vi "parser.vi"() -> ()   [LabVIEW 2009]
uses:
  <vilib>/Utility/file.llb/Read From Spreadsheet File (string).vi
  Global Test Variables DPT.vi
panel:
  out "Header":string[](array[string])
  out "all rows":string[][](array[string])
  out "File Data Out":string[][](array[string])
  in  "OK":bool
  out "array":string[][](array[string])
  out "search string":string
  out "Search for first column data":string
  in  "file path (dialog if empty)":path=path "c:/test1/test.csv"
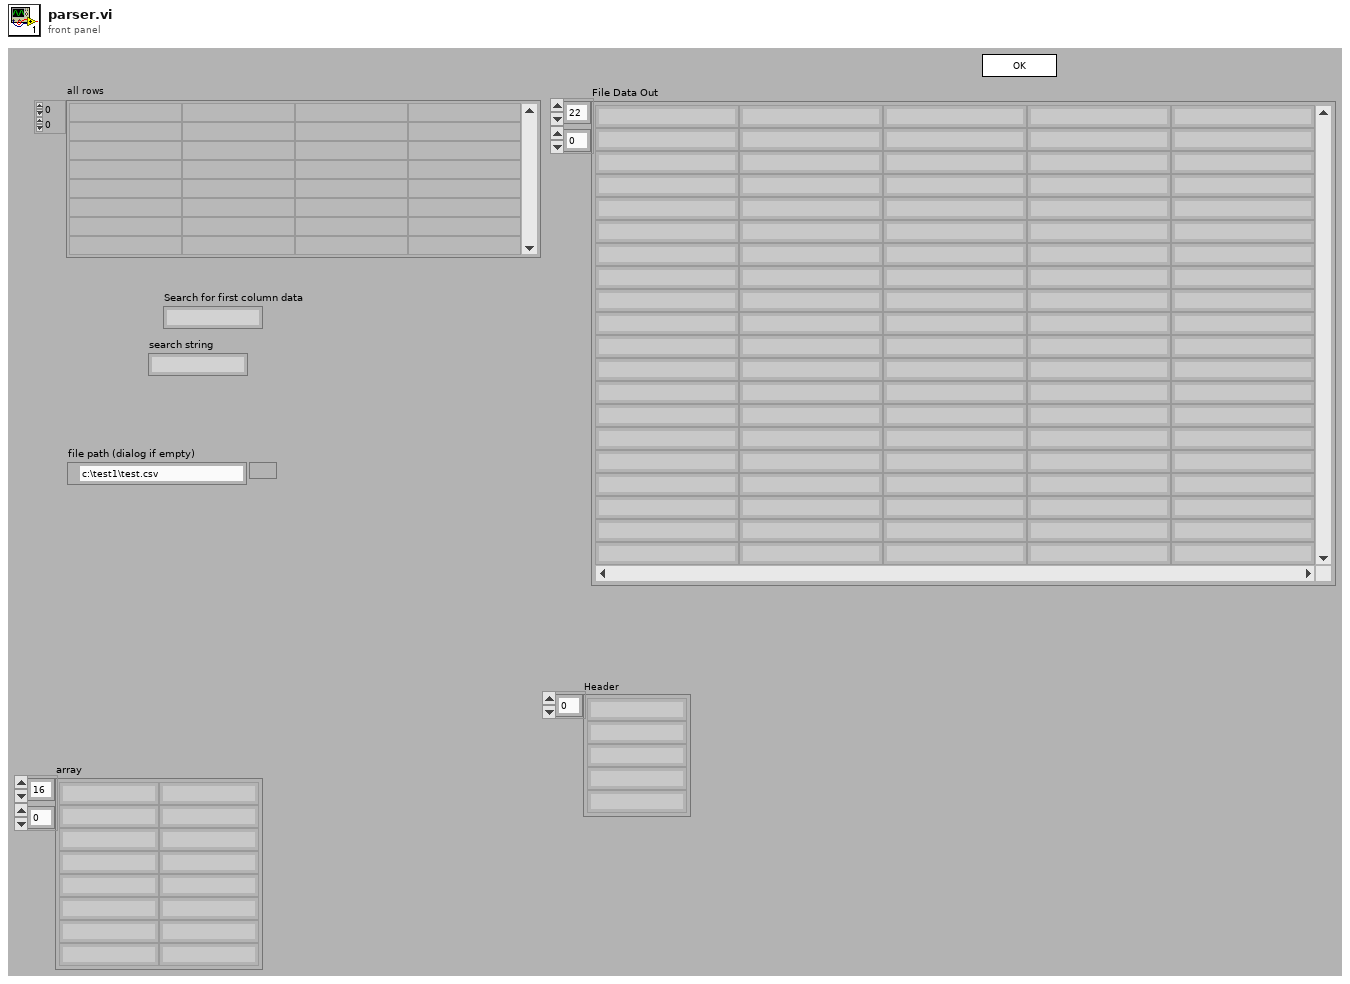
[diagram p1: front panel]
types:
  T1 = enum32{"invalid app kind", "Development System", "Run Time System", "Student Edition", "Embedded LabVIEW", "Evaluation", "Custom"}
  T2 = enum32{"Invalid", "Standard", "Closed", "Hidden", "Minimized", "Maximized"}
  T3 = cluster{"Core":cluster{"Current VI Reference":refnum<vi>, "Close Panel on Exit?":bool}, "File Data In":string[][], "file path (dialog if empty)":path, "File Data Out":string[][], "Header Labels":string[], "Data":dbl[][]}
  T4 = cluster{"Current VI Reference":refnum<vi>, "Close Panel on Exit?":bool}
  T5 = typedef "DOE Audit Data.ctl" = cluster{"Technician":string, "Date":string, "Model":string, "Serial":string, "Total Dry Time(m)":dbl, "Bone Dry Wt":dbl, "Initial Wt":dbl, "Final Wt":dbl, "Initial Ret":dbl, "Final Ret":dbl, "Elect Energy Used":dbl, "Gas Meter Temp":dbl, "Gas Meter Pres":dbl, "Gas Volume":dbl, "Barometer Temp":dbl, "Barometer Pres":dbl, "Gas Corr Fact":dbl, "Cor Gas Vol":dbl, "Gas Heat Val":dbl, "Gas Energy BTU":dbl, "Gas Energy kwh":dbl, "Total Energy":dbl, "4% adjust Energy":dbl, "Gas Vol Init":dbl, "Gas Vol Fin":dbl, "Start Time(s)":dbl, "End Time(s)":dbl, "Elect Energy Start":dbl, "Elect Energy End":dbl, "Per Cycle Efficency":dbl, "Annual Consumption":dbl, "Load Cycles":string, "Ambinet Temp":string, "Ambinet RH":string}
  T6 = cluster{"Initial Wt":dbl, "Final Wt":dbl, "Initial Ret":dbl, "Final Ret":dbl}
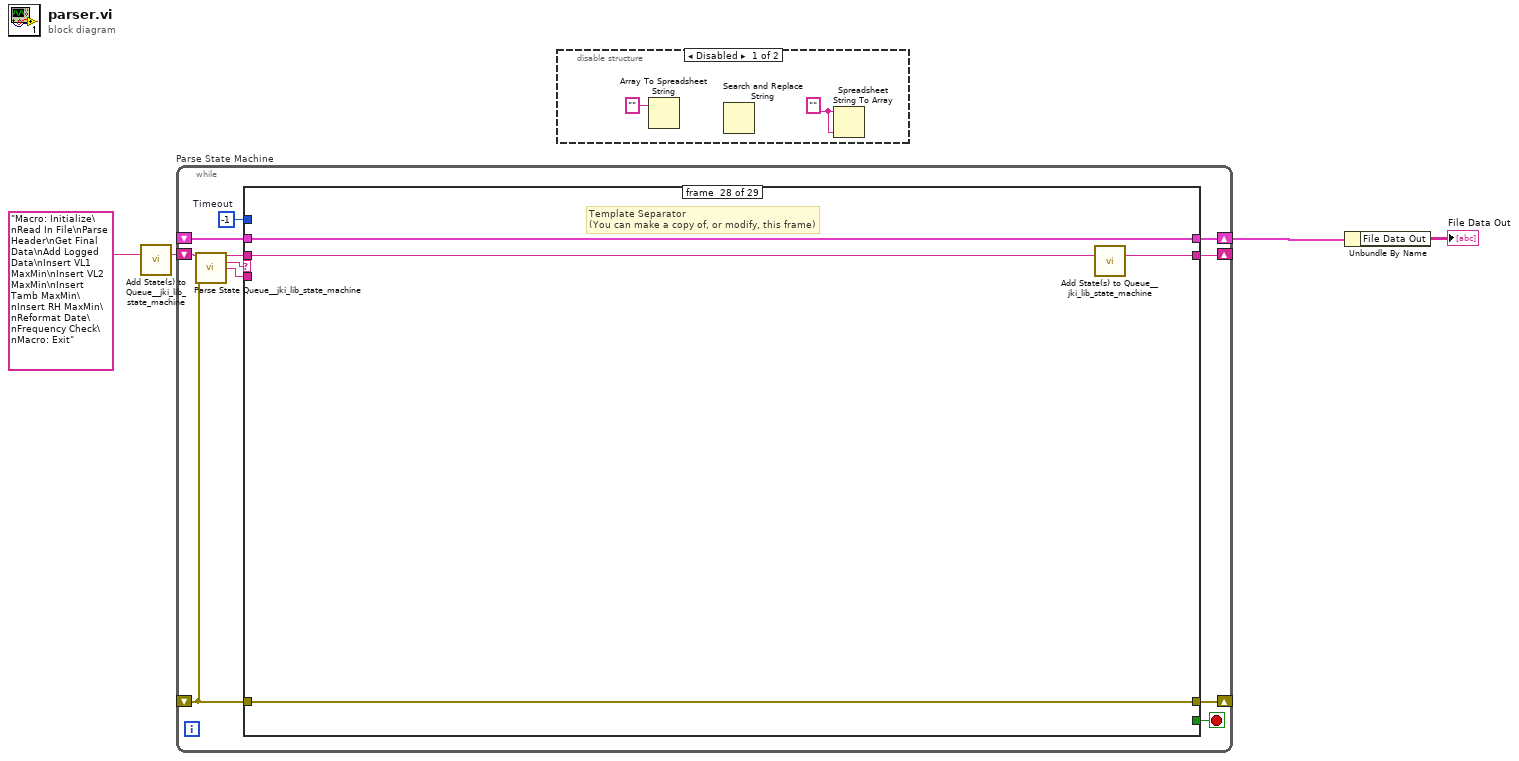
[diagram p0: block diagram]
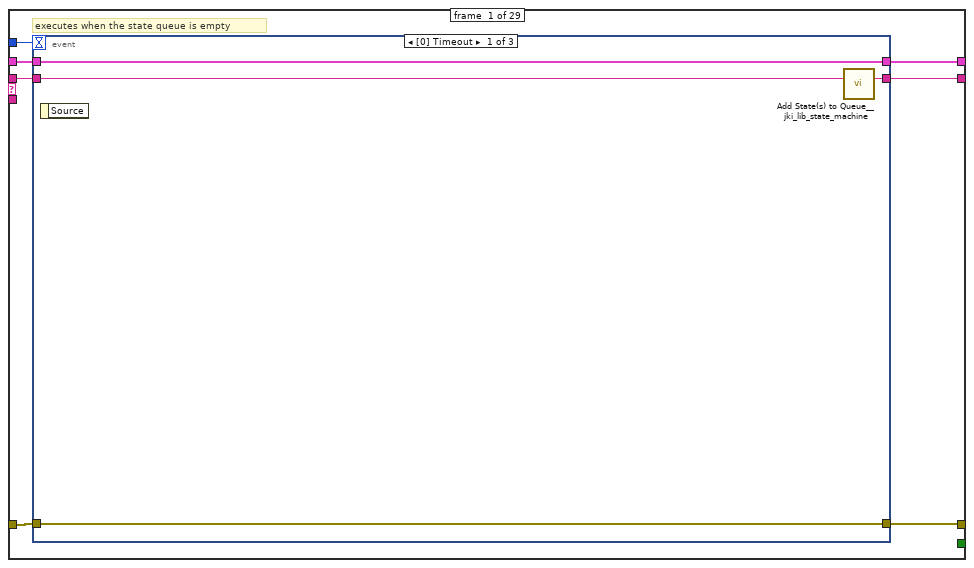
[diagram p3: hidden frame]
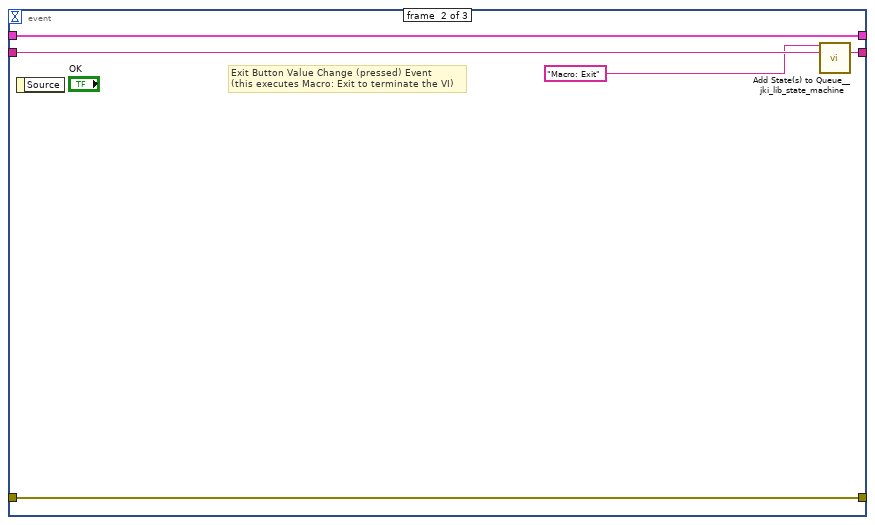
[diagram p4: hidden frame]
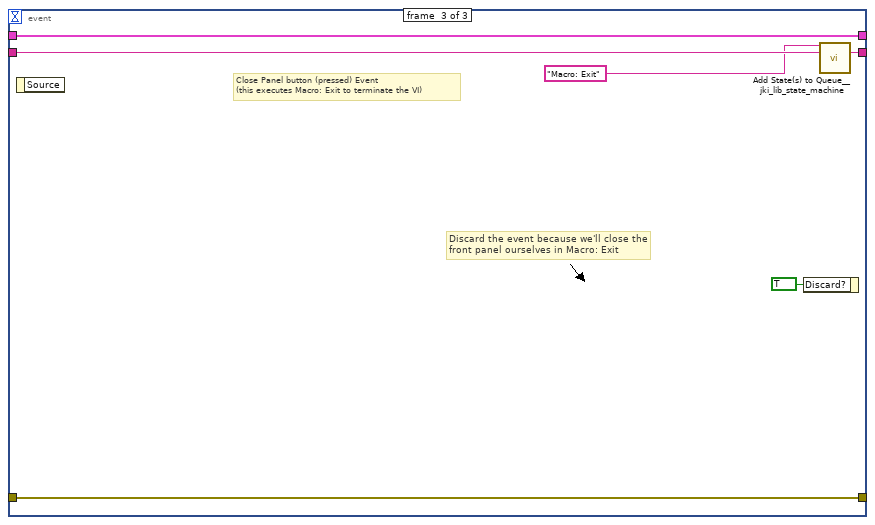
[diagram p5: hidden frame]
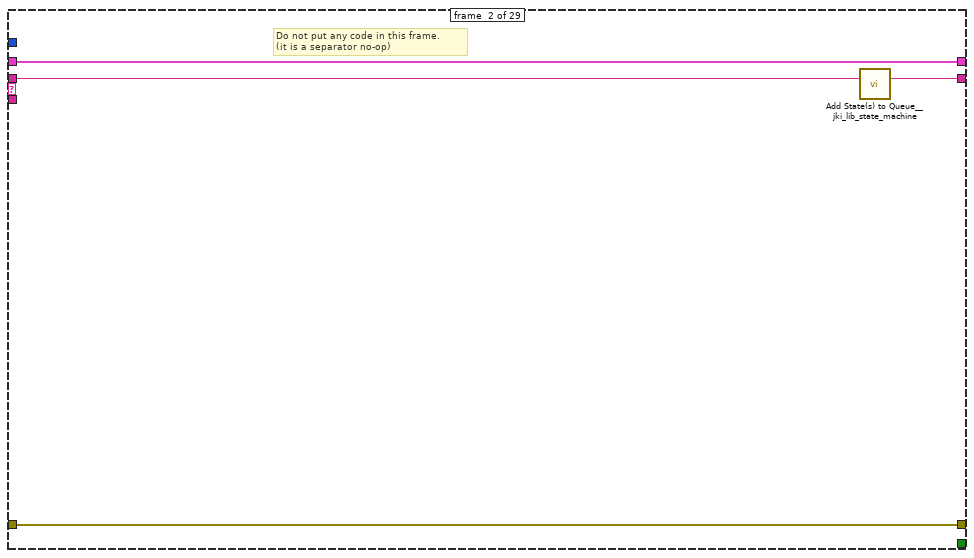
[diagram p6: hidden frame]
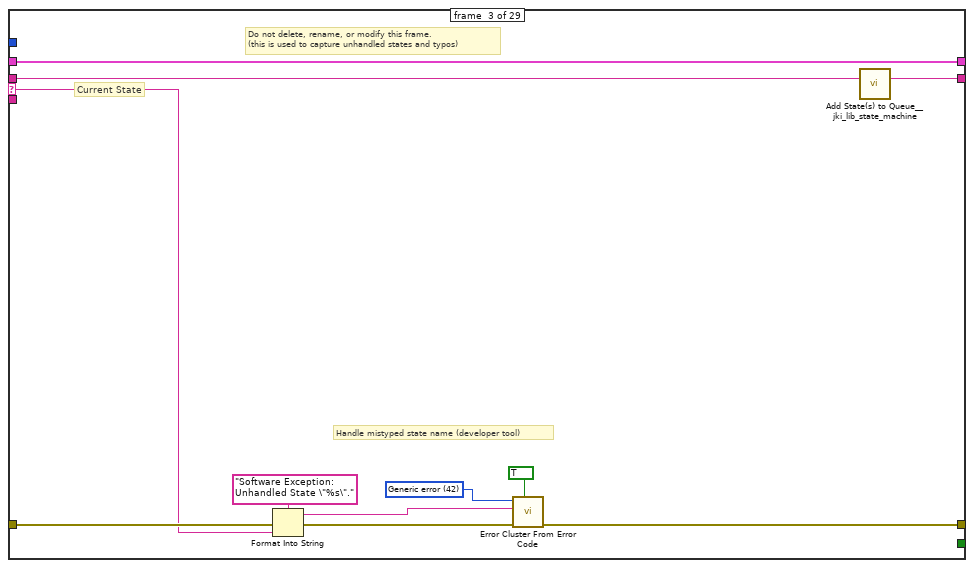
[diagram p7: hidden frame]
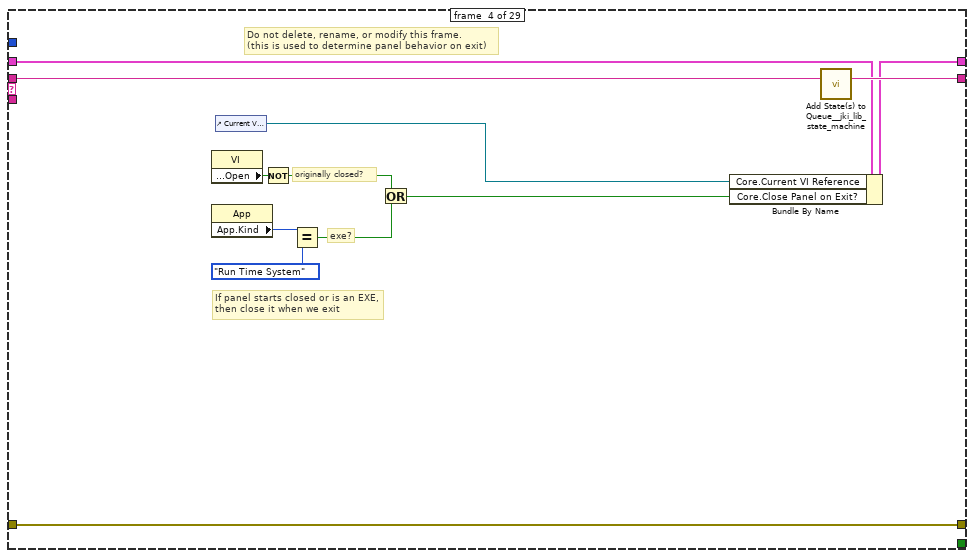
[diagram p8: hidden frame]
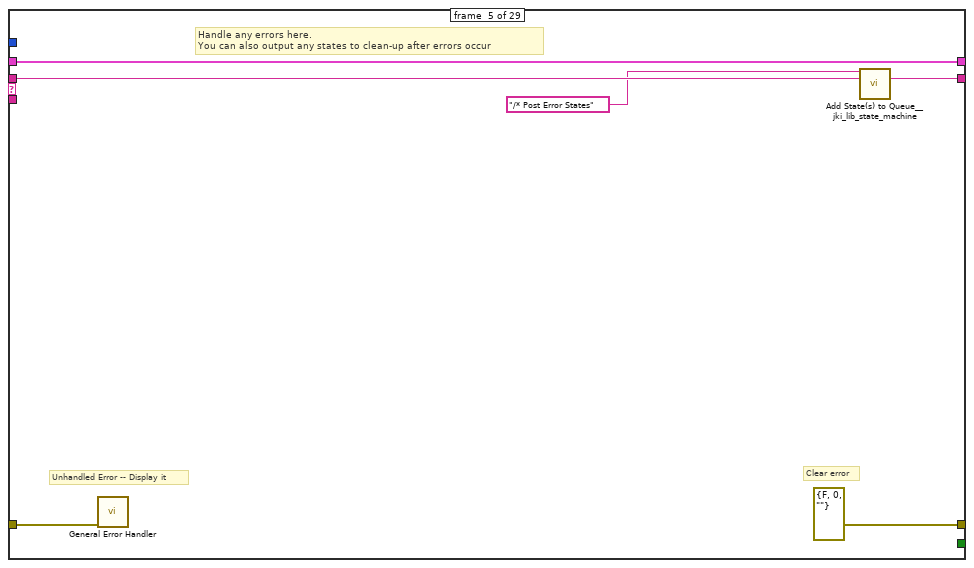
[diagram p9: hidden frame]
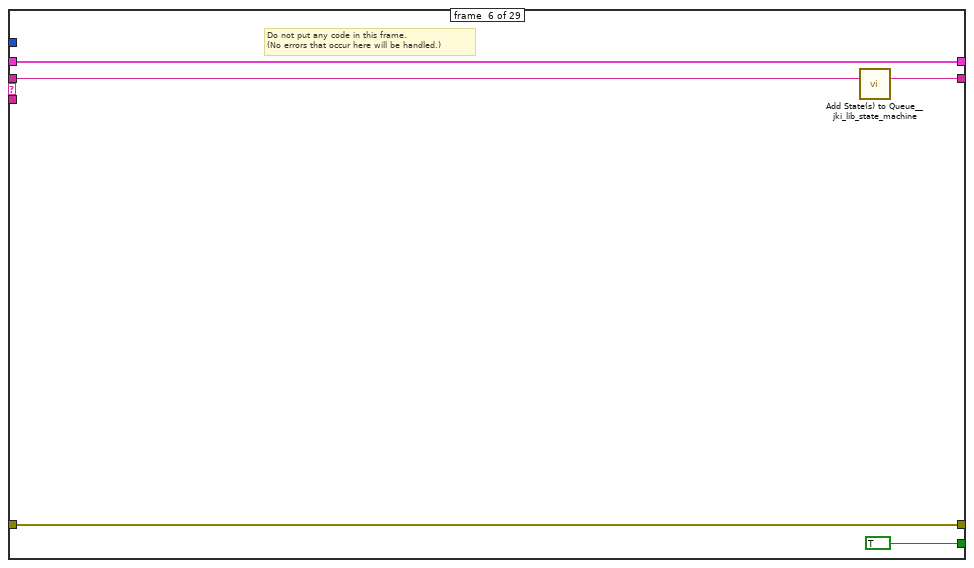
[diagram p10: hidden frame]
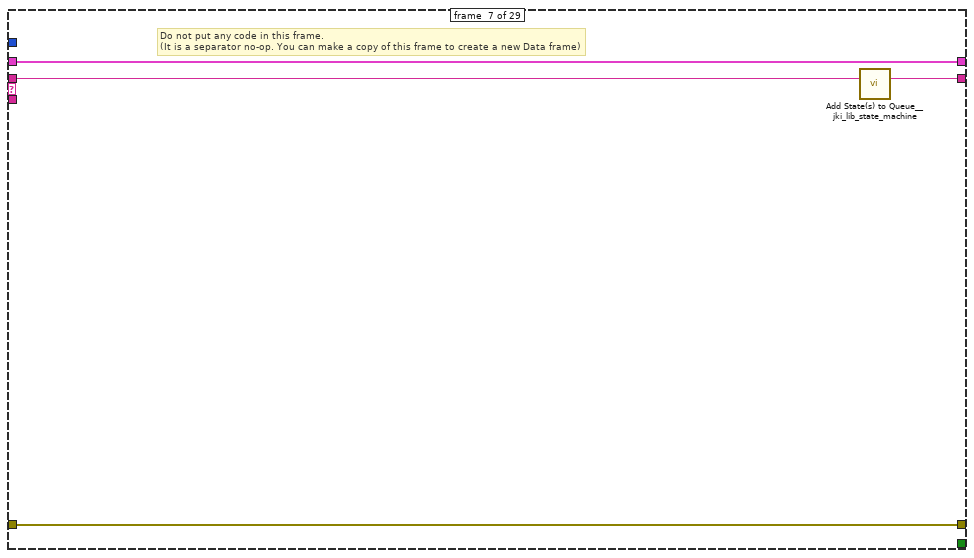
[diagram p11: hidden frame]
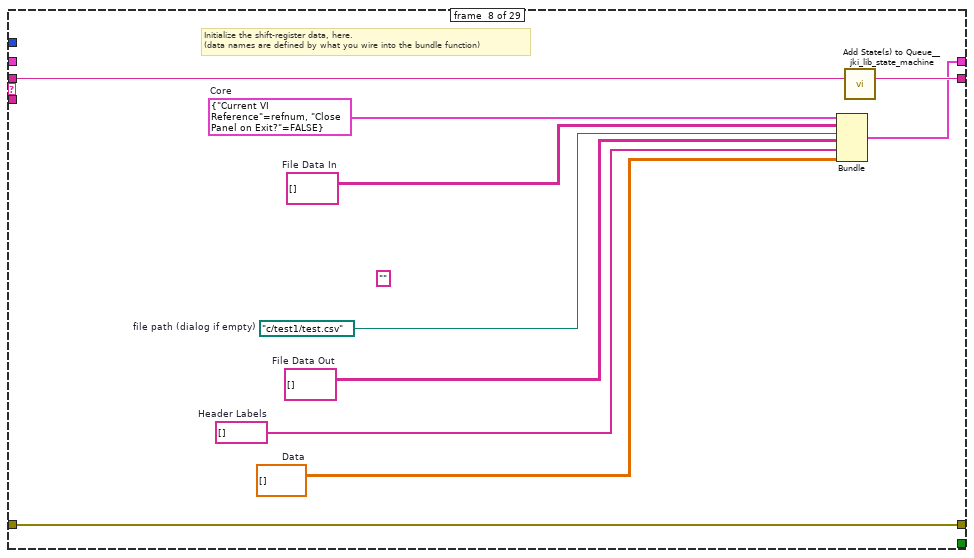
[diagram p12: hidden frame]
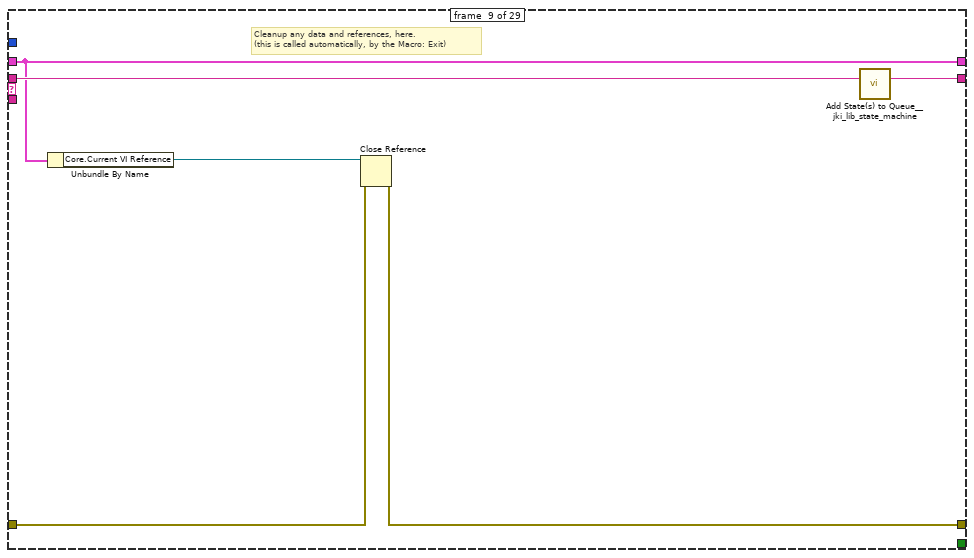
[diagram p13: hidden frame]
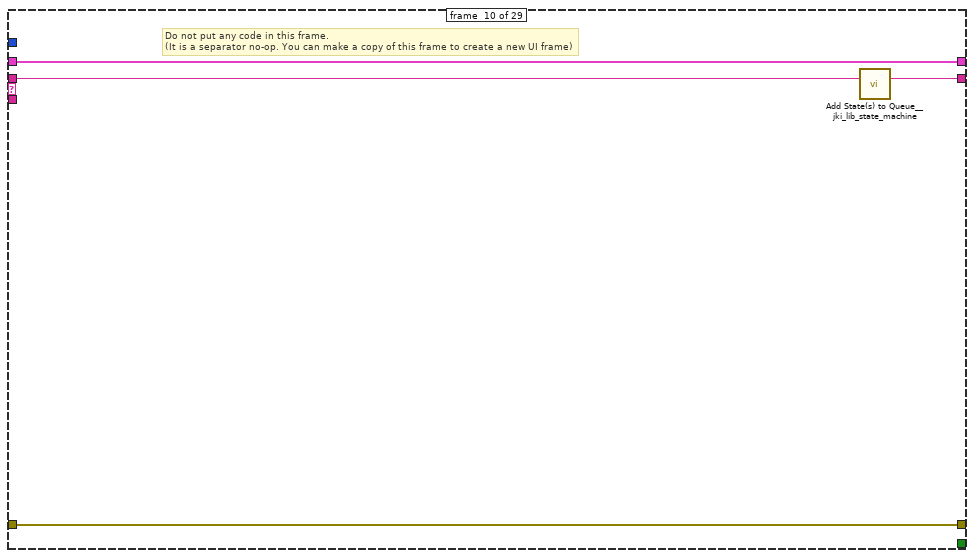
[diagram p14: hidden frame]
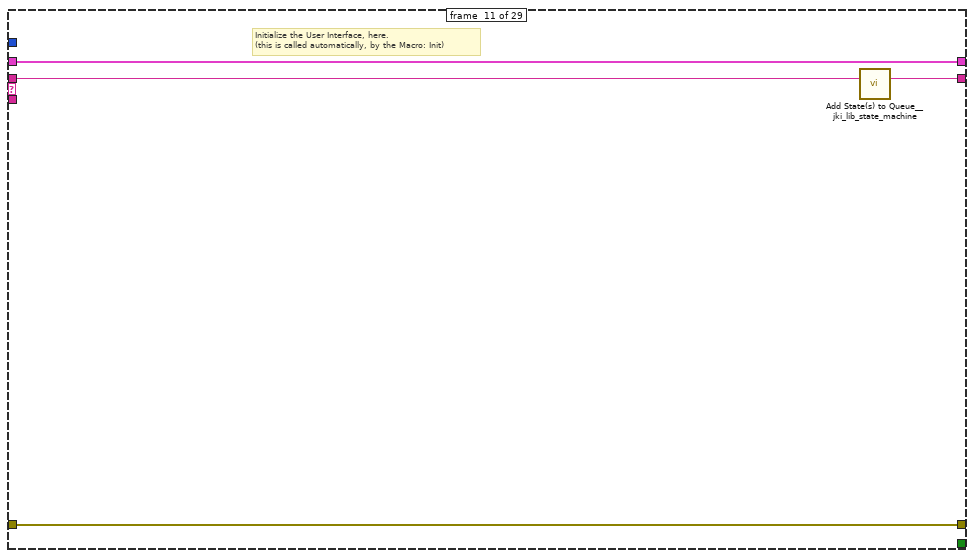
[diagram p15: hidden frame]
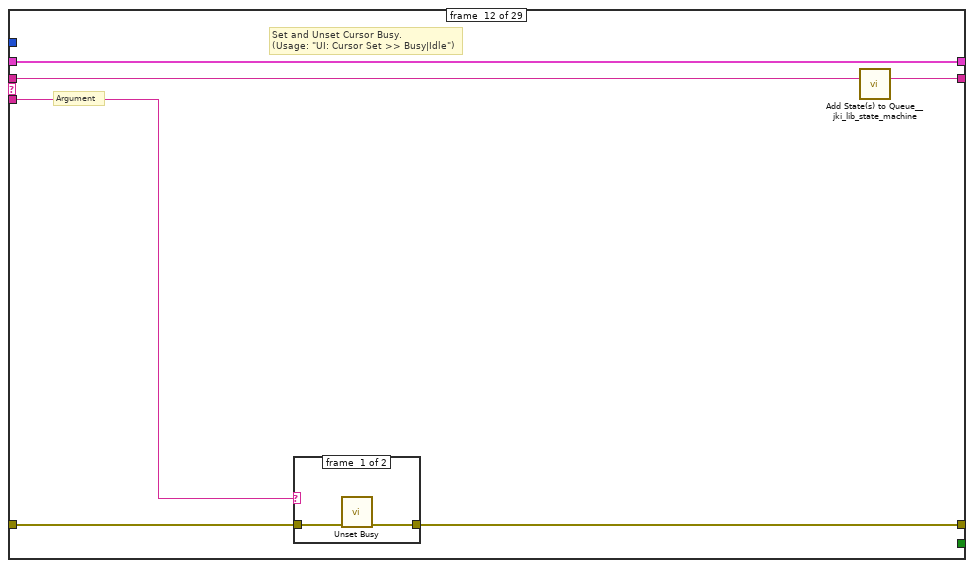
[diagram p16: hidden frame]
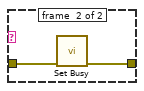
[diagram p17: hidden frame]
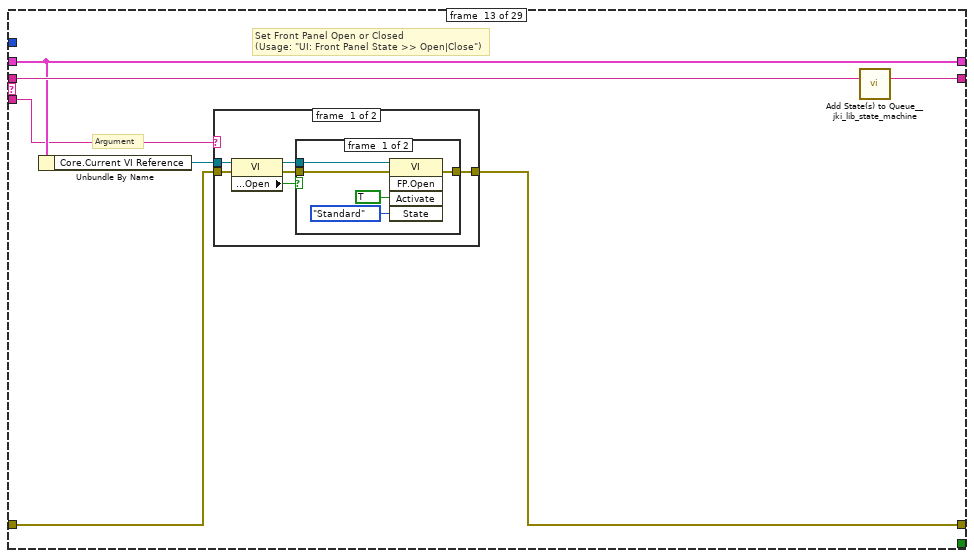
[diagram p18: hidden frame]
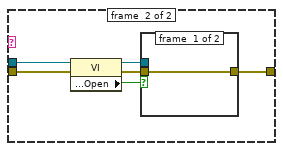
[diagram p20: hidden frame]
diagram:
  n1 = call <vilib>:"Add State(s) to Queue__jki_lib_state_machine.vi"("State(s) in (\"\")"="Macro: Initialize\nRead In File\nParse Header\nGet Final Data\nAdd Logged Data\nInsert VL1 MaxMin\nInsert VL2 MaxMin\nInsert Tamb MaxMin\nInsert RH MaxMin\nReformat Date\nFrequency Check\nMacro: Exit") -> ("States Out"=w4:string)  [unwired: 14 in]
  n2 = while "Parse State Machine" {
    shift-right: [w8] -> w2
    shift-left: _ -> [w7]
    shift-right: [w11] -> _
    shift-left: _ -> [w5]
    shift-right: [w10] -> _
    shift-left: w4 -> [w12]
    stop <- w9 stop-if-true
    w6 = -1  # Timeout
    n3 = call <vilib>:"Parse State Queue__jki_lib_state_machine.vi"("State Queue"=w12, "Error In (no error)"=w5) -> ("Remaining States"=w14:string, "Current State"=w15:string, "Arguments"=w13:string)  [unwired: 11 in]
    n4 = case shown="\"Get Final Data\"" w15 {
      selector: w15 -> [_ _ w42 _ _ _ _ _ _ _ _ _ _ _ _ _ _ _ _ _ _ _ _ _ _ _ _ _ _]
      tunnel: w14 -> [w22 w41 w46 w64 w70 w75 w79 w89 w95 w99 w103 w109 w120 w146 w151 w161 w165 w173 w190 w227 w249 w315 w341 w367 w393 w415 w430 w440 w454]
      tunnel: w13 -> [_ _ _ _ _ _ _ _ _ _ _ w104 w114 _ _ _ _ _ _ _ _ _ _ _ _ _ _ _ w444]
      tunnel: w7 -> [w20 w38 w44 w55 w67 w73 w76 _ w90 w96 w101 w107 w116 w143 w148 w158 w162 w168 w177 w212 w246 w297 w323 w349 w375 w395 w421 w437 w451]
      tunnel: [w19 w39 w48 w61 errorcluster {"status"=FALSE, "code"=0, "source"=""} ("error out") w72 w77 w86 w91 w97 w100 w105 w117 w144 w149 w159 w163 w171 w188 w225 w247 w313 w339 w365 w391 w413 w428 w438 w452] -> w11
      tunnel: w5 -> [w18 w39 w47 w61 w66 w72 w77 w86 w92 w97 w100 w106 w118 w144 w149 w159 w163 w171 w188 w225 w247 w313 w339 w365 w391 w413 w428 w438 w452]
      tunnel: [w21 w40 w45 w63 w69 w74 w78 w88 w94 w98 w102 w108 w119 w145 w150 w160 w164 w172 w189 w226 w248 w314 w340 w366 w392 w414 w429 w439 w453] -> w10
      tunnel: [_ _ _ _ _ TRUE _ _ _ _ _ _ _ _ _ _ _ _ _ _ _ _ _ _ _ _ _ _ _] -> w9
      tunnel: [w17 w38 w44 w62 w67 w73 w76 w87 w90 w96 w101 w107 w116 w143 w148 w158 w162 w167 w176 w211 w245 w297 w323 w349 w375 w396 w422 w437 w450] -> w8
      tunnel: w6 -> [w16 _ _ _ _ _ _ _ _ _ _ _ _ _ _ _ _ _ _ _ _ _ _ _ _ _ _ _ _]
      frame #0 {
        # "executes when the state queue is empty"
        n5 = event shown="[0] Timeout" {
          selector: _ -> [_ _ _]
          dyn-events: _ -> [_ _ _]
          timeout: w16 -> [_ _ _]
          tunnel: w22 -> [w26 w31 w37]
          tunnel: [w25 w30 w36] -> w21
          tunnel: w20 -> [w23 w28 w34]
          tunnel: [w24 w29 w35] -> w19
          tunnel: w18 -> [w24 w29 w35]
          tunnel: [w23 w28 w34] -> w17
          event #0 {
            n6 = event-data() -> ()  [unwired: 1 in, 1 out]
            n7 = call <vilib>:"Add State(s) to Queue__jki_lib_state_machine.vi"("State(s) in (\"\")"=w26) -> ("States Out"=w25:string)  [unwired: 14 in]
          }
          event #1 {
            # "Exit Button Value Change (pressed) Event\n(this executes Macro: Exit to terminate the VI)"
            n8 = event-data() -> ()  [unwired: 1 in, 1 out]
            n9 = call <vilib>:"Add State(s) to Queue__jki_lib_state_machine.vi"("State(s) in Front (\"\")"="Macro: Exit", "State(s) in (\"\")"=w31) -> ("States Out"=w30:string)  [unwired: 13 in]
          }
          event #2 {
            # "Discard the event because we'll close the front panel ourselves in Macro: Exit"
            # "Close Panel button (pressed) Event\n(this executes Macro: Exit to terminate the VI)"
            n10 = event-data() -> ()  [unwired: 1 in, 1 out]
            n11 = event-data("Discard?"=TRUE) -> ()  [unwired: 1 in, 1 out]
            n12 = call <vilib>:"Add State(s) to Queue__jki_lib_state_machine.vi"("State(s) in Front (\"\")"="Macro: Exit", "State(s) in (\"\")"=w37) -> ("States Out"=w36:string)  [unwired: 13 in]
          }
        }
      }
      frame #1 {
        # "Do not put any code in this frame.\n(it is a separator no-op)"
        n13 = call <vilib>:"Add State(s) to Queue__jki_lib_state_machine.vi"("State(s) in (\"\")"=w41) -> ("States Out"=w40:string)  [unwired: 14 in]
      }
      frame #2 {
        w51 = 42 items=["No error", "Argument error", "Memory is full", "Out of zone", "End of file", "File already open", "Generic file I/O error", "File not found", "File permission error", "Disk is full", "Duplicate path", "Too many files open", "System feature not enabled", "Resource file not found", "Cannot add resource", "Resource not found", "Image not found", "Image memory error", "Pen does not exist", "Config type invalid", "Config token not found", "Config parse error", "Config memory error", "Bad external code format", "Bad external code offset", "External code not present", "Null window", "Destroy window error", "Null menu", "Print aborted", "Bad print record", "Print driver error", "Windows error during printing", "Memory error during printing", "Print dialog error", "Generic print error", "Invalid device refnum", "Device not found", "Device parameter error", "Device unit error", "Cannot open device", "Device call aborted", "Generic error", "Cancelled by user", "Object ID too low", "Object ID too high", "Object not in heap", "Unknown heap", "Unknown object (invalid DefProc)", "Unknown object (DefProc not in table)", "Message out of range", "Invalid (null) method", "Unknown message", "Manager call not supported", "Bad address", "Network operation in progress", "Network operation timed out", "Connection is busy", "Network attribute not supported", "Network error", "Address in use", "System out of memory", "Connection aborted", "Connection refused", "Not connected", "Already connected", "Connection closed", "Initialization error (interapplication manager)", "Bad occurrence", "Wait on unbound occurrence handler", "Occurrence queue overflow", "Datalog type conflict", "Unused", "Unrecognized type (interapplication manager)", "Memory corrupt", "Failed to make temporary DLL", "Old CIN version", "Drag socket not found", "Failed to load drop-object", "Failed to register OLE object", "Failed to release OLE object", "Format specifier type mismatch", "Unknown format specifier", "Too few format specifiers", "Too many format specifiers", "Scan failed", "Newer CIN version", "Error converting to variant", "Runtime menu error", "Password tampered", "Variant attribute not found", "Incompatible variant data type", "Event data is not available", "Event Store is not present", "Occurrence is not found", "Event Queue is not created", "Event info is not available", "Refnum passed is NULL", "Error retrieving Class GUID", "Error retrieving CoClass GUID", "Error retrieving TypeLib GUID.", "Bad built application magic bytes.", "Specific driver is different from the specific driver associated with the Logical Name.", "There is no session opened to the class driver.", "Max Error", "MAX - Error with config objects", "MAX - Error loading configuration", "MAX - Group not supported"]
        # "Current State"
        # "Do not delete, rename, or modify this frame.\n(this is used to capture unhandled states and typos)"
        # "Handle mistyped state name (developer tool)"
        n14 = Format Into String(format string="Software Exception: Unhandled State \"%s\"." ("message"), error in=w47, w42) -> (resulting string=w50:string, error out=w49:errorcluster)  [unwired: 1 in]
        n15 = call <vilib>:"Error Cluster From Error Code.vi"("show call chain? (False)"=TRUE, "error in (no error)"=w49, "error message (\"\")"=w50, "error code (0)"=w51) -> ("error out"=w48:errorcluster)  [unwired: 5 in]
        n16 = call <vilib>:"Add State(s) to Queue__jki_lib_state_machine.vi"("State(s) in (\"\")"=w46) -> ("States Out"=w45:string)  [unwired: 14 in]
      }
      frame #3 {
        # "Do not delete, rename, or modify this frame.\n(this is used to determine panel behavior on exit)"
        # "originally closed?"
        # "exe?"
        # "If panel starts closed or is an EXE, then close it when we exit"
        n17 = property class="VI"() -> ("Front Panel.Open"=w60:bool)  [unwired: 2 in, 2 out]
        n18 = property class="App"() -> ("App.Kind"=w59:T1)  [unwired: 2 in, 2 out]
        n19 = control-ref of="Current VI Reference"() -> (w53:refnum<vi>)
        n20 = Not(x=w60) -> (.not. x?=w57:bool)
        n21 = Equal?(x=w59, y=T1."Run Time System" ("Application:Kind")) -> (x = y?=w56:bool)
        n22 = Or(x=w57, y=w56) -> (x .or. y?=w54:bool)
        n23 = Bundle By Name(cluster=w55, "Core.Current VI Reference"=w53, "Core.Close Panel on Exit?"=w54) -> (w62:T3)
        n24 = call <vilib>:"Add State(s) to Queue__jki_lib_state_machine.vi"("State(s) in (\"\")"=w64) -> ("States Out"=w63:string)  [unwired: 14 in]
      }
      frame #4 {
        # "Unhandled Error -- Display it"
        # "Handle any errors here.\nYou can also output any states to clean-up after errors occur"
        # "Clear error"
        n25 = call <vilib>:"General Error Handler.vi"("error in (no error)"=w66) -> ()  [unwired: 10 in, 5 out]
        n26 = call <vilib>:"Add State(s) to Queue__jki_lib_state_machine.vi"("State(s) in Front (\"\")"="/* Post Error States", "State(s) in (\"\")"=w70) -> ("States Out"=w69:string)  [unwired: 13 in]
      }
      frame #5 {
        # "Do not put any code in this frame.\n(No errors that occur here will be handled.)"
        n27 = call <vilib>:"Add State(s) to Queue__jki_lib_state_machine.vi"("State(s) in (\"\")"=w75) -> ("States Out"=w74:string)  [unwired: 14 in]
      }
      frame #6 {
        # "Do not put any code in this frame.\n(It is a separator no-op. You can make a copy of this frame to create a new Data frame)"
        n28 = call <vilib>:"Add State(s) to Queue__jki_lib_state_machine.vi"("State(s) in (\"\")"=w79) -> ("States Out"=w78:string)  [unwired: 14 in]
      }
      frame #7 {
        (unwired) "" ("String")
        w80 = dbl[][] []  # Data
        w81 = string[] []  # Header Labels
        w82 = string[][] []  # File Data Out
        w83 = path "c:/test1/test.csv"  # file path (dialog if empty)
        w84 = string[][] []  # File Data In
        w85 = T4 {"Current VI Reference"=refnum, "Close Panel on Exit?"=FALSE}  # Core
        # "Initialize the shift-register data, here.\n(data names are defined by what you wire into the bundle function)"
        n29 = Bundle("Core"=w85, "File Data In"=w84, "file path (dialog if empty)"=w83, "File Data Out"=w82, "Header Labels"=w81, "Data"=w80) -> (w87:T3)  [unwired: 1 in]
        n30 = call <vilib>:"Add State(s) to Queue__jki_lib_state_machine.vi"("State(s) in (\"\")"=w89) -> ("States Out"=w88:string)  [unwired: 14 in]
      }
      frame #8 {
        # "Cleanup any data and references, here.\n(this is called automatically, by the Macro: Exit)"
        n31 = Unbundle By Name(w90) -> ("Core.Current VI Reference"=w93:refnum<vi>)
        n32 = Close Reference(reference=w93, error in (no error)=w92) -> (error out=w91:errorcluster)
        n33 = call <vilib>:"Add State(s) to Queue__jki_lib_state_machine.vi"("State(s) in (\"\")"=w95) -> ("States Out"=w94:string)  [unwired: 14 in]
      }
      frame #9 {
        # "Do not put any code in this frame.\n(It is a separator no-op. You can make a copy of this frame to create a new UI frame)"
        n34 = call <vilib>:"Add State(s) to Queue__jki_lib_state_machine.vi"("State(s) in (\"\")"=w99) -> ("States Out"=w98:string)  [unwired: 14 in]
      }
      frame #10 {
        # "Initialize the User Interface, here.\n(this is called automatically, by the Macro: Init)"
        n35 = call <vilib>:"Add State(s) to Queue__jki_lib_state_machine.vi"("State(s) in (\"\")"=w103) -> ("States Out"=w102:string)  [unwired: 14 in]
      }
      frame #11 {
        # "Argument"
        # "Set and Unset Cursor Busy.\n(Usage: \"UI: Cursor Set >> Busy|Idle\")"
        n36 = case shown="\"Idle\", Default" w104 {
          tunnel: w106 -> [w111 w113]
          tunnel: [w110 w112] -> w105
          frame #0 {
            n37 = call <vilib>:"Unset Busy.vi"("error in (no error)"=w111) -> ("error out"=w110:errorcluster)  [unwired: 10 in]
          }
          frame #1 {
            n38 = call <vilib>:"Set Busy.vi"("error in (no error)"=w113) -> ("error out"=w112:errorcluster)  [unwired: 9 in, 1 out]
          }
        }
        n39 = call <vilib>:"Add State(s) to Queue__jki_lib_state_machine.vi"("State(s) in (\"\")"=w109) -> ("States Out"=w108:string)  [unwired: 14 in]
      }
      frame #12 {
        # "Argument"
        # "Set Front Panel Open or Closed\n(Usage: \"UI: Front Panel State >> Open|Close\")"
        n40 = Unbundle By Name(w116) -> ("Core.Current VI Reference"=w115:refnum<vi>)
        n41 = case shown="\"Open\", Default" w114 {
          tunnel: w118 -> [w124 w137]
          tunnel: [w126 w138] -> w117
          tunnel: w115 -> [w125 w135]
          frame #0 {
            n42 = property class="VI"(reference=w125, error in=w124) -> (reference out=w122:refnum<vi>, error out=w123:errorcluster, "Front Panel.Open"=w121:bool)
            n43 = case shown="False" w121 {
              tunnel: [w129 w132] -> w126
              tunnel: w123 -> [w128 w132]
              tunnel: w122 -> [w127 _]
              frame #0 {
                n44 = invoke class="VI" method="FP.Open"(reference=w127, error in=w128, "Activate"=TRUE, "State"=T2."Standard") -> (error out=w129:errorcluster)  [unwired: 1 in, 4 out]
              }
              frame #1 {
              }
            }
          }
          frame #1 {
            n45 = property class="VI"(reference=w135, error in=w137) -> (reference out=w134:refnum<vi>, error out=w136:errorcluster, "Front Panel.Open"=w133:bool)
            n46 = case shown="True" w133 {
              tunnel: [w139 w142] -> w138
              tunnel: w136 -> [w139 w141]
              tunnel: w134 -> [_ w140]
              frame #0 {
              }
              frame #1 {
                n47 = invoke class="VI" method="FP.Close"(reference=w140, error in=w141) -> (error out=w142:errorcluster)  [unwired: 1 in, 2 out]
              }
            }
          }
        }
        n48 = call <vilib>:"Add State(s) to Queue__jki_lib_state_machine.vi"("State(s) in (\"\")"=w120) -> ("States Out"=w119:string)  [unwired: 14 in]
      }
      frame #13 {
        # "Do not put any code in this frame.\n(It is a separator no-op. You can make a copy of this frame to create a new Macro frame)"
        n49 = call <vilib>:"Add State(s) to Queue__jki_lib_state_machine.vi"("State(s) in (\"\")"=w146) -> ("States Out"=w145:string)  [unwired: 14 in]
      }
      frame #14 {
        w147 = "Data: Initialize\nInitialize Core Data\nUI: Initialize\nUI: Front Panel State >> Open"  # Data: Initialize Initialize Core Data UI: Initialize UI: Front Panel State >> Open
        # "Initialization Macro\n(This is called once, when the VI starts)"
        n50 = call <vilib>:"Add State(s) to Queue__jki_lib_state_machine.vi"("State(s) in Front (\"\")"=w147, "State(s) in (\"\")"=w151) -> ("States Out"=w150:string)  [unwired: 13 in]
      }
      frame #15 {
        # "Exit Macro\n(This is called once, when the VI exits)"
        n51 = Unbundle By Name(w158) -> ("Core.Close Panel on Exit?"=w157:bool)
        n52 = Select(t="UI: Front Panel State >> Close", s=w157, f="") -> (s? t:f=w154:string)
        n53 = call <vilib>:"Add State(s) to Queue__jki_lib_state_machine.vi"("State(s) in (\"\")"=w154, "State(s) at Back (\"\")"="Data: Cleanup\nExit") -> ("States Out"=w152:string)  [unwired: 13 in]
        n54 = call <vilib>:"Add State(s) to Queue__jki_lib_state_machine.vi"("State(s) in Front (\"\")"=w152, "State(s) in (\"\")"=w161) -> ("States Out"=w160:string)  [unwired: 13 in]
      }
      frame #16 {
        # "Template Separator\n(You can make a copy of, or modify, this frame)"
        n55 = call <vilib>:"Add State(s) to Queue__jki_lib_state_machine.vi"("State(s) in (\"\")"=w165) -> ("States Out"=w164:string)  [unwired: 14 in]
      }
      frame #17 {
        n56 = call-poly <vilib>:"Read From Spreadsheet File.vi"("delimiter (\\t)"="," ("delimiter (\\t)"), "file path (dialog if empty)"="file path (dialog if empty)") -> ("all rows"=w166:string[][])  [unwired: 5 in, 4 out]
        "all rows" <- w166
        n57 = Bundle By Name(cluster=w168, "File Data In"=w166) -> (w167:T3)
        n58 = call <vilib>:"Add State(s) to Queue__jki_lib_state_machine.vi"("State(s) in (\"\")"=w173) -> ("States Out"=w172:string)  [unwired: 14 in]
      }
      frame #18 {
        w178 = "TEST STATION:\t&Station \nCOMPUTER_NAME:\t&Computername\nVERSION:\t&Version\nTR_NUMBER:\t&TR#\nENGINEER:\t&Engineer\nTECHNICIAN:\t&Tech\nFILENAME:\t&Filename\nCOMMENTS:\t&Comments\nDATE:\t&Date\nBuild\t&Build\nLAB ID:\t&Unit\nMODEL:\t&Model\nSerial Number\t&Serial\nSerial Number\t&Dryer Type\nSUPPLY VOLTAGE:\t&Voltage\nFrequency:\t&Freq\nDrum Volume\t&Volume\nTEST_TYPE:\t&Test Type\nTEST_TITLE:\t&Title\nTEST NUM:\t&Test Number\nNom Load Type\t&Load Type\nNom Load Weight\t&Load Size\nLOAD RUN NUM:\t&Run\nDRYING CYCLE:\t&Drying Cycle\nHeat Setting\t&Heat Setting\nDryness Setting\t&Dryness setting\nEXHAUST:\t&Restriction\nBone Dry Wt\t&BDW\n"  # Label, replace string
        w187 = "" ("format string")
        w179 = "" ("format string")
        w184 = "STATION / NAME:\t&Station / &Computername\nVERSION:\t&Version\n--------------------------\t--------------------------\nTR #:\t&TR#\nENGINEER:\t&Engineer\nTECHNICIAN:\t&Tech\n--------------------------\t--------------------------\nFILENAME:\t&Filename\nCOMMENTS:\t&Comments\nDATE:\t&Date\n--------------------------\t--------------------------\nBUILD:\t&Build\nUNIT:\t&Unit\nMODEL #:\t&Model\nSERIAL #:\t&Serial\nDRYER TYPE:\t&Dryer Type\nSUPPLY VOLTAGE:\t&Voltage\nFREQUENCY (Hz):\t&Freq\nDRUM VOL (cuft):\t&Volume\n--------------------------\t--------------------------\nTEST TYPE:\t&Test Type\nTEST TITLE:\t&Title\nTEST #:\t&Test Numver\nLOAD TYPE:\t&Load Type\nLOAD SIZE (lbs):\t&Load Size\nLOAD RUN #:\t&Run\n--------------------------\t--------------------------\nDRYING CYCLE:\t&Drying Cycle\nHEAT SETTING:\t&Heat Setting\nDRYNESS SETTING:\t&Dryness setting\nRESTRICTION:\t&Restriction\nBONE DRY WT (lbs):\t&BDW\nINITIAL WT (lbs):\t&InitWeight\nFINAL WT (lbs):\t&FinalWeight\nIMC:\t&IMC\nFMC:\t&FMC\nFMC DELAY (min):\t&FMCDelay\n--------------------------\t--------------------------\nAMB TEMP (F):\t&AmbTemp\nAMB RH (%):\t&RH\nAMB TEMP (Max / Min):\t&TempMaxMin\nAMB RH (Max / Min):\t&RHMaxMin\nVOLTAGE L1 (Max / Min):\t&VL1MaxMin\nVOLTAGE L2 (Max / Min):\t&VL2MaxMin\n--------------------------\t--------------------------\n"  # ProtoData
        # "Your code here.\n(You can make a copy of, or modify, this frame)"
        n59 = Unbundle By Name(w177) -> ("File Data In"=w175:string[][])
        n60 = local write "File Data Out"(w175) -> ()
        n61 = Delete From Array(array=w175, index (col)=0 ("disabled index (col)")) -> (deleted portion=w181:string[])  [unwired: 2 in, 1 out]
        n62 = Delete From Array(array=w175, index (col)=1 ("disabled index (col)")) -> (deleted portion=w183:string[])  [unwired: 2 in, 1 out]
        n63 = Spreadsheet String To Array(format string=w179, spreadsheet string=w178, array type (2D Dbl)=w179) -> (array=w185:string[][])  [unwired: 1 in]
        "array" <- w185
        n64 = for {
          tunnel: w181 -> [w201]
          tunnel: w183 -> [w199]
          tunnel: w185 -> [w196] mode=indexing
          shift-right: [w191] -> w186
          shift-left: w184 -> [w198]
          n65 = Index Array(array=w196, index #1=0 ("index"), index #2=1 ("index")) -> (element #1=w193:string, element #2=w192:string)
          "Search for first column data" <- w193
          "search string" <- w192
          n66 = Search 1D Array(1D array=w201, element=w193) -> (index of element=w200:i32)  [unwired: 1 in]
          n67 = Index Array(array=w199, index=w200) -> (element=w197:string)
          n68 = Search and Replace String(input string=w198, search string=w192, replace string=w197) -> (result string=w191:string)  [unwired: 5 in, 3 out]
        }
        n69 = Spreadsheet String To Array(format string=w187, spreadsheet string=w186, array type (2D Dbl)=w187) -> (array=w174:string[][])  [unwired: 1 in]
        n70 = Bundle By Name(cluster=w177, "File Data Out"=w174) -> (w176:T3)
        n71 = local write "File Data Out"(w174) -> ()
        n72 = call <vilib>:"Add State(s) to Queue__jki_lib_state_machine.vi"("State(s) in (\"\")"=w190) -> ("States Out"=w189:string)  [unwired: 14 in]
      }
      frame #19 {
        w206 = "" ("format string")
        # "Your code here.\n(You can make a copy of, or modify, this frame)"
        n73 = call "Worksheet DOE Audit.vi"() -> ("DOE Data Out"=w224:T5)  [unwired: 9 in, 1 out]
        n74 = Unbundle By Name(w212) -> ("File Data Out"=w208:string[][])
        n75 = Unbundle By Name(w224) -> ("Initial Wt"=w223:dbl, "Final Wt"=w220:dbl, "Initial Ret"=w221:dbl, "Final Ret"=w222:dbl, "Ambinet Temp"=w203:string, "Ambinet RH"=w202:string)
        n76 = Bundle("Initial Wt"=w223, "Final Wt"=w220, "Initial Ret"=w221, "Final Ret"=w222) -> (w219:T6)  [unwired: 1 in]
        n77 = Cluster To Array(cluster=w219) -> (array=w218:dbl[])
        n78 = Array To Spreadsheet String(array=w208, 3:"" ("format string")) -> (spreadsheet string=w209:string)  [unwired: 1 in]
        n79 = Number To Fractional String(number=w218, precision (6)=i16 1) -> (F-format string=w216:string[])  [unwired: 2 in]
        n80 = call "String2Array.vi"("Delimiter"="\\n", "String"="&InitWeight\n&FinalWeight\n&IMC\n&FMC\n&AmbTemp\n&RH") -> ("Array"=w215:string[])  [unwired: 9 in]
        n81 = Build Array (concatenate)(w216, w203, w202) -> (w204:string[])
        n82 = for {
          tunnel: w215 -> [w229] mode=indexing
          shift-right: [w230] -> w210
          shift-left: w209 -> [w231]
          tunnel: w204 -> [w228] mode=indexing
          n83 = Search and Replace String(input string=w231, search string=w229, replace string=w228) -> (result string=w230:string)  [unwired: 5 in, 3 out]
        }
        n84 = Spreadsheet String To Array(format string=w206, spreadsheet string=w210, array type (2D Dbl)=w206) -> (array=w205:string[][])  [unwired: 1 in]
        n85 = call <vilib>:"Add State(s) to Queue__jki_lib_state_machine.vi"("State(s) in (\"\")"=w227) -> ("States Out"=w226:string)  [unwired: 14 in]
        n86 = Bundle By Name(cluster=w212, "File Data Out"=w205) -> (w211:T3)
        n87 = local write "File Data Out"(w205) -> ()
      }
      frame #20 {
        # "Add the data after the header"
        # "Your code here.\n(You can make a copy of, or modify, this frame)"
        n88 = global read "Global Test Variables DPT.vi" "Header Search Key2"() -> (w233:string)
        n89 = global read "Global Test Variables DPT.vi" "Header Search Key1"() -> (w234:string)
        n90 = Unbundle By Name(w246) -> ("File Data In"=w241:string[][], "File Data Out"=w236:string[][])
        n91 = Index Array(array=w241, index (col)=0 ("disabled index (col)")) -> (element=w232:string[])  [unwired: 1 in]
        n92 = Search 1D Array(1D array=w232, element=w234) -> (index of element=w238:i32)  [unwired: 1 in]
        n93 = Search 1D Array(1D array=w232, element=w233) -> (index of element=w237:i32)  [unwired: 1 in]
        n94 = Greater Than 0?(x=w238) -> (x > 0?=w239:bool)
        n95 = Greater Than 0?(x=w237) -> (x > 0?=w242:bool)
        n96 = Exclusive Or(1:w242, 2:w239) -> (0:w243:bool)
        n97 = Select(t=w238, s=w239, f=w237) -> (s? t:f=w235:i32)
        n98 = case shown="True" w243 {
          tunnel: w246 -> [w253 w289]
          tunnel: [w252 w288] -> w245
          tunnel: w241 -> [w251 w287]
          tunnel: ["Macro: Exit" ("element") _] -> w240
          tunnel: w235 -> [_ w283]
          tunnel: w236 -> [_ w285]
          frame #0 {
            n99 = Bundle By Name(cluster=w253, "File Data Out"=w251) -> (w252:T3)
          }
          frame #1 {
            w262 = 0 ("index")
            w270 = TRUE
            w261 = 1 ("index")
            # "remove end data\nwhere I< on. MSG lines\ngive 0."
            # "Add only the dryer on data.  Dryer is on when \nIL1 > min current (0.1A)"
            n100 = Delete From Array(array=w287, length=w283, index (row)=0) -> (array with subset deleted=w280:string[][])  [unwired: 1 in, 1 out]
            n101 = Delete From Array(array=w280, index (row)=0) -> (deleted portion=w265:string[], array with subset deleted=w259:string[][])  [unwired: 2 in]
            "Header" <- w265
            n102 = global read "Global Test Variables DPT.vi" "Dryer On Min Current"() -> (w255:dbl)
            n103 = global read "Global Test Variables DPT.vi" "IL1 Header"() -> (w278:string)
            n104 = global read "Global Test Variables DPT.vi" "IL2 Header"() -> (w266:string)
            n105 = Search 1D Array(1D array=w265, element=w278) -> (index of element=w277:i32)  [unwired: 1 in]
            n106 = Array Subset(array=w259, index (row)=w262, index (col)=w277, length (col)=w261) -> (w276:string[][])  [unwired: 1 in]
            n107 = Array Size(array=w276) -> (size(s)=w281:i32[])
            n108 = Multiply Array Elements(1:w281) -> (0:w258:i32)
            n109 = Reshape Array(w276, w258) -> (w282:string[])
            n110 = Fract/Exp String To Number(string=w282) -> (number=w257:dbl[])  [unwired: 3 in, 1 out]
            n111 = Search 1D Array(1D array=w265, element=w266) -> (index of element=w260:i32)  [unwired: 1 in]
            n112 = Array Subset(array=w259, index (row)=w262, index (col)=w260, length (col)=w261) -> (w264:string[][])  [unwired: 1 in]
            n113 = Reshape Array(w264, w258) -> (w263:string[])
            n114 = Fract/Exp String To Number(string=w263) -> (number=w256:dbl[])  [unwired: 3 in, 1 out]
            n115 = Add(x=w257, y=w256) -> (x+y=w254:dbl[])
            n116 = Greater?(x=w254, y=w255) -> (0:w272:bool[])
            n117 = Reverse 1D Array(array=w272) -> (reversed array=w271:bool[])
            n118 = Search 1D Array(1D array=w272, element=w270) -> (index of element=w275:i32)  [unwired: 1 in]
            n119 = Search 1D Array(1D array=w271, element=w270) -> (index of element=w268:i32)  [unwired: 1 in]
            n120 = Subtract(x=w258, y=w275) -> (x-y=w269:i32)
            n121 = Subtract(x=w269, y=w268) -> (x-y=w267:i32)
            n122 = Array Subset(array=w259, index (row)=w275, length (row)=w267) -> (w274:string[][])  [unwired: 2 in]
            n123 = Fract/Exp String To Number(string=w274) -> (number=w273:dbl[][])  [unwired: 3 in, 1 out]
            n124 = Build Array (concatenate)(w285, w265, w274) -> (w284:string[][])
            n125 = local write "File Data Out"(w284) -> ()
            n126 = Bundle By Name(cluster=w289, "File Data Out"=w284, "Header Labels"=w265, "Data"=w273) -> (w288:T3)
          }
        }
        n127 = call <vilib>:"Add State(s) to Queue__jki_lib_state_machine.vi"("State(s) in Front (\"\")"=w240, "State(s) in (\"\")"=w249) -> ("States Out"=w248:string)  [unwired: 13 in]
      }
      frame #21 {
        w294 = "&VL1MaxMin"  # replacement term
        w310 = i16 1 ("precision (6)")
        # "column of term"
        # "These are the elements in column 0 to indicate where\nthe header for the data is."
        # "Your code here.\n(You can make a copy of, or modify, this frame)"
        n128 = Unbundle By Name(w297) -> ("Data"=w299:dbl[][], "Header Labels"=w301:string[])
        n129 = global read "Global Test Variables DPT.vi" "VL1 Header"() -> (w304:string)
        n130 = Array Size(array=w299) -> (size(s)=w312:i32[])
        n131 = Search 1D Array(1D array=w301, element=w304) -> (index of element=w303:i32)  [unwired: 1 in]
        n132 = Index Array(array=w312, index=0) -> (element=w300:i32)
        n133 = Array Subset(array=w299, length (row)=w300, index (col)=w303, length (col)=1 ("length")) -> (w298:dbl[][])  [unwired: 1 in]
        n134 = Array Max & Min(array=w298) -> (max value=w306:dbl, min value=w305:dbl)  [unwired: 2 out]
        n135 = Number To Fractional String(number=w306, precision (6)=w310) -> (F-format string=w309:string)  [unwired: 2 in]
        n136 = Number To Fractional String(number=w305, precision (6)=w310) -> (F-format string=w307:string)  [unwired: 2 in]
        n137 = Concatenate Strings(w309, "/" ("string"), w307) -> (w291:string)
        n138 = Search and Replace String(input string="Replace Data Out Term >> xxx,yyy" ("State(s) in Front (\"\")"), search string="xxx", replace string=w294) -> (result string=w292:string)  [unwired: 5 in, 3 out]
        n139 = Search and Replace String(input string=w292, search string="yyy", replace string=w291) -> (result string=w290:string)  [unwired: 5 in, 3 out]
        n140 = call <vilib>:"Add State(s) to Queue__jki_lib_state_machine.vi"("State(s) in Front (\"\")"=w290, "State(s) in (\"\")"=w315) -> ("States Out"=w314:string)  [unwired: 13 in]
      }
      frame #22 {
        w320 = "&VL2MaxMin"  # replacement term
        w336 = i16 1 ("precision (6)")
        # "column of term"
        # "These are the elements in column 0 to indicate where\nthe header for the data is."
        # "Your code here.\n(You can make a copy of, or modify, this frame)"
        n141 = Unbundle By Name(w323) -> ("Data"=w325:dbl[][], "Header Labels"=w327:string[])
        n142 = global read "Global Test Variables DPT.vi" "VL2 Header"() -> (w330:string)
        n143 = Array Size(array=w325) -> (size(s)=w338:i32[])
        n144 = Search 1D Array(1D array=w327, element=w330) -> (index of element=w329:i32)  [unwired: 1 in]
        n145 = Index Array(array=w338, index=0) -> (element=w326:i32)
        n146 = Array Subset(array=w325, length (row)=w326, index (col)=w329, length (col)=1 ("length")) -> (w324:dbl[][])  [unwired: 1 in]
        n147 = Array Max & Min(array=w324) -> (max value=w332:dbl, min value=w331:dbl)  [unwired: 2 out]
        n148 = Number To Fractional String(number=w332, precision (6)=w336) -> (F-format string=w335:string)  [unwired: 2 in]
        n149 = Number To Fractional String(number=w331, precision (6)=w336) -> (F-format string=w333:string)  [unwired: 2 in]
        n150 = Concatenate Strings(w335, "/" ("string"), w333) -> (w317:string)
        n151 = Search and Replace String(input string="Replace Data Out Term >> xxx,yyy" ("State(s) in Front (\"\")"), search string="xxx", replace string=w320) -> (result string=w318:string)  [unwired: 5 in, 3 out]
        n152 = Search and Replace String(input string=w318, search string="yyy", replace string=w317) -> (result string=w316:string)  [unwired: 5 in, 3 out]
        n153 = call <vilib>:"Add State(s) to Queue__jki_lib_state_machine.vi"("State(s) in Front (\"\")"=w316, "State(s) in (\"\")"=w341) -> ("States Out"=w340:string)  [unwired: 13 in]
      }
      frame #23 {
        w346 = "&TempMaxMin"  # replacement term
        w362 = i16 1 ("precision (6)")
        # "column of term"
        # "These are the elements in column 0 to indicate where\nthe header for the data is."
        # "Your code here.\n(You can make a copy of, or modify, this frame)"
        n154 = Unbundle By Name(w349) -> ("Data"=w351:dbl[][], "Header Labels"=w353:string[])
        n155 = global read "Global Test Variables DPT.vi" "Tambient Header"() -> (w356:string)
        n156 = Array Size(array=w351) -> (size(s)=w364:i32[])
        n157 = Search 1D Array(1D array=w353, element=w356) -> (index of element=w355:i32)  [unwired: 1 in]
        n158 = Index Array(array=w364, index=0) -> (element=w352:i32)
        n159 = Array Subset(array=w351, length (row)=w352, index (col)=w355, length (col)=1 ("length")) -> (w350:dbl[][])  [unwired: 1 in]
        n160 = Array Max & Min(array=w350) -> (max value=w358:dbl, min value=w357:dbl)  [unwired: 2 out]
        n161 = Number To Fractional String(number=w358, precision (6)=w362) -> (F-format string=w361:string)  [unwired: 2 in]
        n162 = Number To Fractional String(number=w357, precision (6)=w362) -> (F-format string=w359:string)  [unwired: 2 in]
        n163 = Concatenate Strings(w361, "/" ("string"), w359) -> (w343:string)
        n164 = Search and Replace String(input string="Replace Data Out Term >> xxx,yyy" ("State(s) in Front (\"\")"), search string="xxx", replace string=w346) -> (result string=w344:string)  [unwired: 5 in, 3 out]
        n165 = Search and Replace String(input string=w344, search string="yyy", replace string=w343) -> (result string=w342:string)  [unwired: 5 in, 3 out]
        n166 = call <vilib>:"Add State(s) to Queue__jki_lib_state_machine.vi"("State(s) in Front (\"\")"=w342, "State(s) in (\"\")"=w367) -> ("States Out"=w366:string)  [unwired: 13 in]
      }
      frame #24 {
        w372 = "&RHMaxMin"  # replacement term
        w388 = i16 1 ("precision (6)")
        # "column of term"
        # "These are the elements in column 0 to indicate where\nthe header for the data is."
        # "Your code here.\n(You can make a copy of, or modify, this frame)"
        n167 = Unbundle By Name(w375) -> ("Data"=w377:dbl[][], "Header Labels"=w379:string[])
        n168 = global read "Global Test Variables DPT.vi" "RH Header"() -> (w382:string)
        n169 = Array Size(array=w377) -> (size(s)=w390:i32[])
        n170 = Search 1D Array(1D array=w379, element=w382) -> (index of element=w381:i32)  [unwired: 1 in]
        n171 = Index Array(array=w390, index=0) -> (element=w378:i32)
        n172 = Array Subset(array=w377, length (row)=w378, index (col)=w381, length (col)=1 ("length")) -> (w376:dbl[][])  [unwired: 1 in]
        n173 = Array Max & Min(array=w376) -> (max value=w384:dbl, min value=w383:dbl)  [unwired: 2 out]
        n174 = Number To Fractional String(number=w384, precision (6)=w388) -> (F-format string=w387:string)  [unwired: 2 in]
        n175 = Number To Fractional String(number=w383, precision (6)=w388) -> (F-format string=w385:string)  [unwired: 2 in]
        n176 = Concatenate Strings(w387, "/" ("string"), w385) -> (w369:string)
        n177 = Search and Replace String(input string="Replace Data Out Term >> xxx,yyy" ("State(s) in Front (\"\")"), search string="xxx", replace string=w372) -> (result string=w370:string)  [unwired: 5 in, 3 out]
        n178 = Search and Replace String(input string=w370, search string="yyy", replace string=w369) -> (result string=w368:string)  [unwired: 5 in, 3 out]
        n179 = call <vilib>:"Add State(s) to Queue__jki_lib_state_machine.vi"("State(s) in Front (\"\")"=w368, "State(s) in (\"\")"=w393) -> ("States Out"=w392:string)  [unwired: 13 in]
      }
      frame #25 {
        w402 = "-"
        w407 = 1  # column of Date Data
        # "These are the elements in column 0 to indicate where\nthe header for the data is."
        # "Your code here.\n(You can make a copy of, or modify, this frame)"
        n180 = Unbundle By Name(w395) -> ("File Data Out"=w409:string[][])
        n181 = Index Array(array=w409, index (col)=0 ("disabled index (col)")) -> (element=w411:string[])  [unwired: 1 in]
        n182 = global read "Global Test Variables DPT.vi" "Date Label"() -> (w410:string)
        n183 = Search 1D Array(1D array=w411, element=w410) -> (index of element=w408:i32)  [unwired: 1 in]
        n184 = Index Array(array=w409, index (row)=w408, index (col)=w407) -> (element=w405:string)
        n185 = Scan From String(format string="%4s%2s%2s%3s%2s", input string=w405) -> (output 1=w404:string, output 2=w403:string, output 3=w400:string, output 4=w399:string, output 5=w398:string)  [unwired: 7 in, 3 out]
        n186 = Concatenate Strings(w404, w402, w403, w402, w400, w399, ":" ("string"), w398) -> (w397:string)
        n187 = Replace Array Subset(array=w409, new element=w397, index (row)=w408, index (col)=w407) -> (w394:string[][])
        n188 = Bundle By Name(cluster=w395, "File Data Out"=w394) -> (w396:T3)
        n189 = call <vilib>:"Add State(s) to Queue__jki_lib_state_machine.vi"("State(s) in (\"\")"=w415) -> ("States Out"=w414:string)  [unwired: 14 in]
      }
      frame #26 {
        w423 = 1  # column of freq Data
        # "These are the elements in column 0 to indicate where\nthe header for the data is."
        # "Your code here.\n(You can make a copy of, or modify, this frame)"
        n190 = Unbundle By Name(w421) -> ("File Data Out"=w424:string[][])
        n191 = Index Array(array=w424, index (col)=0 ("disabled index (col)")) -> (element=w426:string[])  [unwired: 1 in]
        n192 = global read "Global Test Variables DPT.vi" "Frequency Label"() -> (w425:string)
        n193 = Search 1D Array(1D array=w426, element=w425) -> (index of element=w419:i32)  [unwired: 1 in]
        n194 = Index Array(array=w424, index (row)=w419, index (col)=w423) -> (element=w418:string)
        n195 = Equal?(x=w418, y="") -> (x = y?=w416:bool)
        n196 = case shown="False" w416 {
          tunnel: w424 -> [w431 w436]
          tunnel: w423 -> [_ w435]
          tunnel: [w431 w434] -> w420
          tunnel: w419 -> [_ w433]
          frame #0 {
          }
          frame #1 {
            n197 = Replace Array Subset(array=w436, new element="60" ("new element/subarray"), index (row)=w433, index (col)=w435) -> (w434:string[][])
          }
        }
        n198 = Bundle By Name(cluster=w421, "File Data Out"=w420) -> (w422:T3)
        n199 = call <vilib>:"Add State(s) to Queue__jki_lib_state_machine.vi"("State(s) in (\"\")"=w430) -> ("States Out"=w429:string)  [unwired: 14 in]
      }
      frame #27 {
        # "Template Separator\n(You can make a copy of, or modify, this frame)"
        n200 = call <vilib>:"Add State(s) to Queue__jki_lib_state_machine.vi"("State(s) in (\"\")"=w440) -> ("States Out"=w439:string)  [unwired: 14 in]
      }
      frame #28 {
        # "Replace Data Out Term >> &term, value"
        n201 = Match Pattern(string=w444, regular expression=",") -> (before substring=w442:string, after substring=w441:string)  [unwired: 1 in, 2 out]
        n202 = Unbundle By Name(w451) -> ("File Data Out"=w448:string[][])
        n203 = Array To Spreadsheet String(array=w448, 3:"" ("format string")) -> (spreadsheet string=w447:string)  [unwired: 1 in]
        n204 = Search and Replace String(input string=w447, search string=w442, replace string=w441) -> (result string=w446:string)  [unwired: 5 in, 3 out]
        n205 = flat-sequence {
          tunnel: w446 -> [w456]
          tunnel: [w455] -> w445
          frame #0 {
            w457 = "" ("format string")
            n206 = Spreadsheet String To Array(format string=w457, spreadsheet string=w456, array type (2D Dbl)=w457) -> (array=w455:string[][])  [unwired: 1 in]
            n207 = local write "File Data Out"(w455) -> ()
          }
        }
        n208 = Bundle By Name(cluster=w451, "File Data Out"=w445) -> (w450:T3)
        n209 = call <vilib>:"Add State(s) to Queue__jki_lib_state_machine.vi"("State(s) in (\"\")"=w454) -> ("States Out"=w453:string)  [unwired: 14 in]
      }
    }
  }
  n210 = disable-structure shown="Disabled" {
    frame #0 {
      w458 = "" ("format string")
      n211 = Array To Spreadsheet String(3:"" ("format string")) -> ()  [unwired: 2 in, 1 out]
      n212 = Search and Replace String() -> ()  [unwired: 8 in, 4 out]
      n213 = Spreadsheet String To Array(format string=w458, array type (2D Dbl)=w458) -> ()  [unwired: 2 in, 1 out]
    }
    frame #1 {
    }
  }
  n214 = Unbundle By Name(w2) -> ("File Data Out"=→"File Data Out":string[][])
